vi "PbStrobe.vi"(3 "error in (no error)":errorcluster, 5 "VISA resource":refnum<visa-resource-name>="COM1") -> (0 "error out":errorcluster, 2 "dup VISA resource":refnum<visa-resource-name>="COM1")   [LabVIEW 2021]
doc: "Strobes in Pb address\nand data to AVS-47B"
panel:
  # "PbStrobe.vi"
  # "The Picobus Strobe Condition is achieved\nby keeping the clock line CP at zero while\nthe data line from computer DC toggles\nthree cycles. \n   Picobus Strobe must be sent after both \naddress and data."
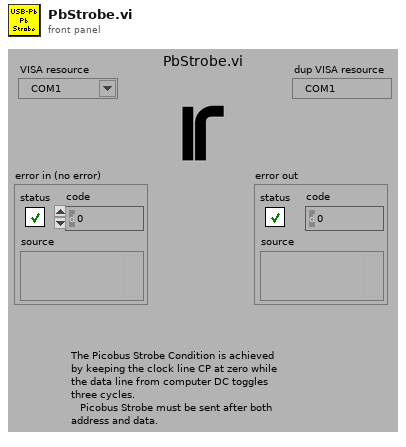
[diagram p1: front panel]
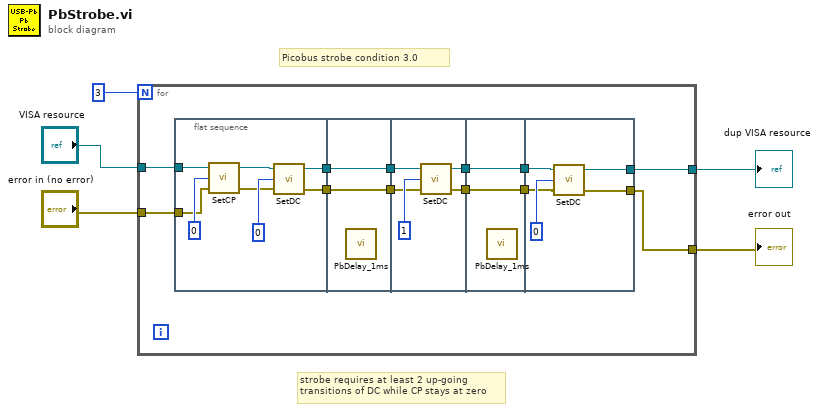
[diagram p0: block diagram]
diagram:
  # "Picobus strobe condition 3.0"
  # "strobe requires at least 2 up-going\ntransitions of DC while CP stays at zero"
  n1 = for {
    N: 3 -> [_]
    tunnel: "VISA resource" -> [w17]
    tunnel: [w12] -> w3
    tunnel: "error in (no error)" -> [w11]
    tunnel: [w6] -> w1
    n2 = flat-sequence {
      tunnel: w17 -> [w25]
      tunnel: [w21] -> w15
      tunnel: w11 -> [w20]
      tunnel: [w18] -> w9
      tunnel: [w27] -> w16
      tunnel: w15 -> [w27]
      tunnel: [w26] -> w10
      tunnel: w9 -> [w26]
      tunnel: w16 -> [w31]
      tunnel: [w30] -> w13
      tunnel: w10 -> [w29]
      tunnel: [w28] -> w7
      tunnel: [w34] -> w14
      tunnel: w13 -> [w34]
      tunnel: [w33] -> w8
      tunnel: w7 -> [w33]
      tunnel: w14 -> [w38]
      tunnel: [w37] -> w12
      tunnel: w8 -> [w36]
      tunnel: [w35] -> w6
      frame #0 {
        n3 = call "SetCP.vi"("error in (no error)"=w20, "CP(=RTS) state"=u8 0, "VISA resource"=w25) -> ("error out"=w19:errorcluster, "dup VISA resource"=w22:refnum<visa-resource-name>)  [unwired: 1 in]
        n4 = call "SetDC.vi"("error in (no error)"=w19, "DC(=DTR) state"=u8 0, "VISA resource"=w22) -> ("error out"=w18:errorcluster, "dup VISA resource"=w21:refnum<visa-resource-name>)  [unwired: 1 in]
      }
      frame #1 {
        n5 = call "PbDelay_1ms.vi"() -> ()  [unwired: 4 in]
      }
      frame #2 {
        n6 = call "SetDC.vi"("error in (no error)"=w29, "DC(=DTR) state"=u8 1, "VISA resource"=w31) -> ("error out"=w28:errorcluster, "dup VISA resource"=w30:refnum<visa-resource-name>)  [unwired: 1 in]
      }
      frame #3 {
        n7 = call "PbDelay_1ms.vi"() -> ()  [unwired: 4 in]
      }
      frame #4 {
        n8 = call "SetDC.vi"("error in (no error)"=w36, "DC(=DTR) state"=u8 0, "VISA resource"=w38) -> ("error out"=w35:errorcluster, "dup VISA resource"=w37:refnum<visa-resource-name>)  [unwired: 1 in]
      }
    }
  }
  "dup VISA resource" <- w3
  "error out" <- w1
